vi "TestExec TCP-IP Listener.Log Manager FG.vi"(7 "Auto Scroll":bool, 9 "Data":string, 10 "Action":enum16{"Init", "Clear", "Log", "Set AutoScroll"}(ring)=enum."Log", 11 "Log":refnum<vi>) -> ()   [LabVIEW 2017]
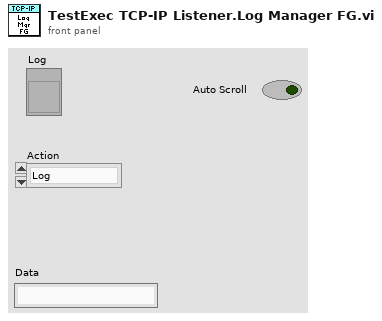
[diagram p1: front panel]
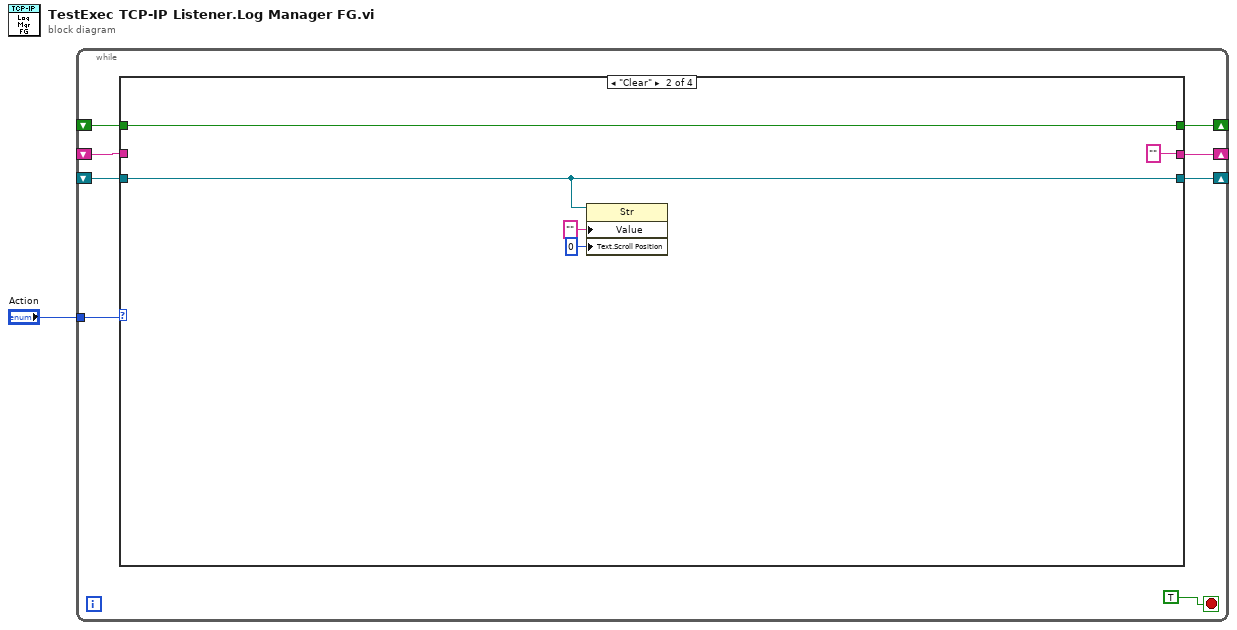
[diagram p0: block diagram]
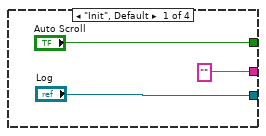
[diagram p2: hidden frame]
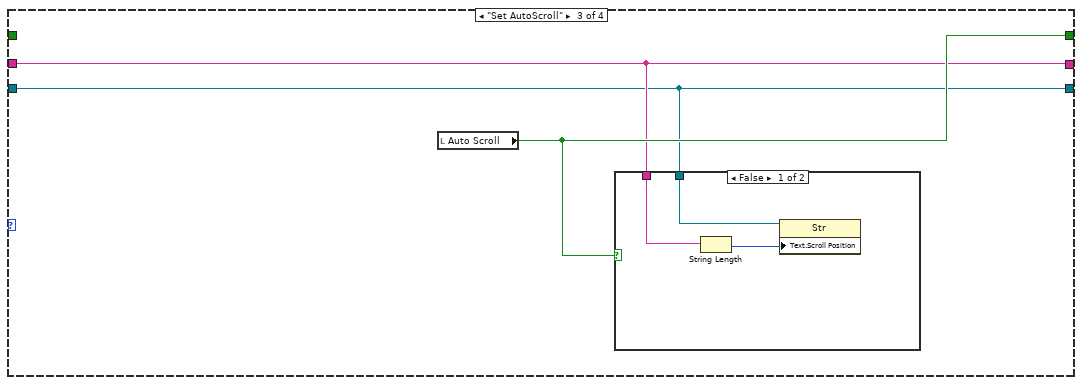
[diagram p3: hidden frame]
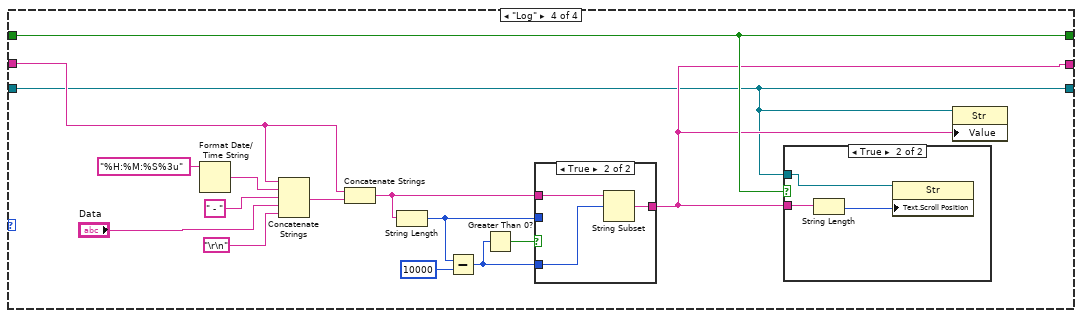
[diagram p5: hidden frame]
diagram:
  n1 = while {
    tunnel: "Action" -> [w9]
    shift-right: [w8] -> _
    shift-left: _ -> [w4]
    shift-right: [w7] -> _
    shift-left: _ -> [w5]
    shift-right: [w6] -> _
    shift-left: _ -> [w3]
    stop <- TRUE stop-if-true
    n2 = case shown="\"Clear\"" w9 {
      tunnel: ["" "" w19 w25] -> w8
      tunnel: ["Auto Scroll" w16 w20 w26] -> w7
      tunnel: ["Log" w15 w18 w24] -> w6
      tunnel: w5 -> [_ w16 _ w26]
      tunnel: w4 -> [_ _ w19 w28]
      tunnel: w3 -> [_ w15 w18 w24]
      frame "Init", Default {
      }
      frame "Clear" {
        n3 = property class="Str"(reference=w15, "Value"="", "Text.Scroll Position"=u32 0) -> ()  [unwired: 1 in, 2 out]
      }
      frame "Set AutoScroll" {
        n4 = local read "Auto Scroll"() -> (w20:bool)
        n5 = case shown="False" w20 {
          tunnel: w19 -> [w21 _]
          tunnel: w18 -> [w22 _]
          frame False {
            n6 = String Length(string=w21) -> (length=w23:i32)
            n7 = property class="Str"(reference=w22, "Text.Scroll Position"=w23) -> ()  [unwired: 1 in, 2 out]
          }
          frame True {
          }
        }
      }
      frame "Log" {
        n8 = Format Date/Time String(time format string (%c)="%H:%M:%S%3u") -> (date/time string=w33:string)  [unwired: 2 in]
        n9 = Concatenate Strings(w28, w33, " - ", "Data", "\r\n") -> (w29:string)
        n10 = Concatenate Strings(w28, w29) -> (w34:string)
        n11 = String Length(string=w34) -> (length=w36:i32)
        n12 = Subtract(x=w36, y=10000) -> (x-y=w35:i32)
        n13 = Greater Than 0?(x=w35) -> (x > 0?=w37:bool)
        n14 = case shown="True" w37 {
          tunnel: w36 -> [_ _]
          tunnel: w35 -> [_ w44]
          tunnel: w34 -> [w42 w45]
          tunnel: [w42 w43] -> w25
          frame False {
          }
          frame True {
            n15 = String Subset(string=w45, offset (0)=w44) -> (substring=w43:string)  [unwired: 1 in]
          }
        }
        n16 = case shown="True" w26 {
          tunnel: w25 -> [_ w41]
          tunnel: w24 -> [_ w40]
          frame False {
          }
          frame True {
            n17 = String Length(string=w41) -> (length=w39:i32)
            n18 = property class="Str"(reference=w40, "Text.Scroll Position"=w39) -> ()  [unwired: 1 in, 2 out]
          }
        }
        n19 = property class="Str"(reference=w24, "Value"=w25) -> ()  [unwired: 1 in, 2 out]
      }
    }
  }
